vi "App.OpenSequenceSettingsFile.vi"(8 "error in (no error)":errorcluster, 11 "selected path":path) -> (0 "error out":errorcluster, 3 "Settings":T1)   [LabVIEW 2013, in "Simple Sequence Tools - Shared.lvlib"]
uses:
  Simple Sequence Tools - Shared.lvlib
  Types/Saved.Sequence.ctl
  Types/Channel.Properties.ctl
  Main.Constants.vi
  <vilib>/NI/GXML/_subVIs/GXML Quick Parser/Quick Parser.vi
  <vilib>/NI/GXML/GXML.lvlib
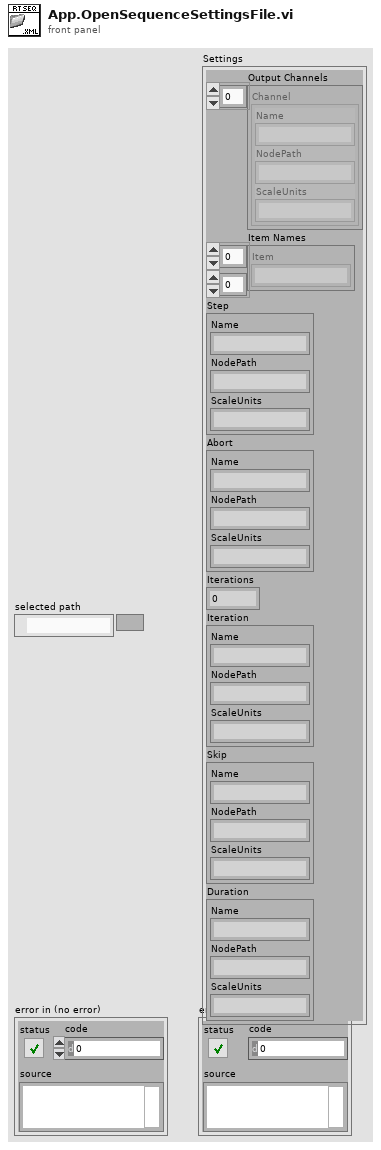
[diagram p1: front panel]
types:
  T1 = typedef "Simple Sequence Tools - Shared.lvlib/Saved.Sequence.ctl" = cluster{"Output Channels":T2[], "Item Names":string[][], "Step":T2, "Abort":T2, "Iterations":u32, "Iteration":T2, "Skip":T2, "Duration":T2}
  T2 = typedef "Simple Sequence Tools - Shared.lvlib/Channel.Properties.ctl" = cluster{"Name":string, "NodePath":string, "ScaleUnits":string}
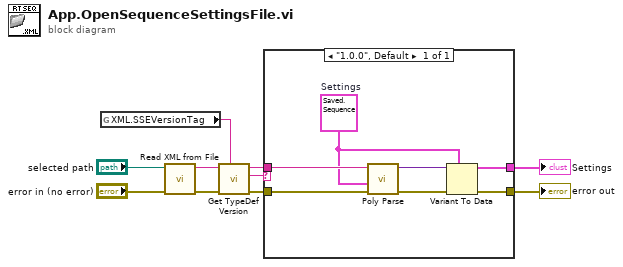
[diagram p0: block diagram]
diagram:
  n1 = global read "Main.Constants.vi" "XML.SSEVersionTag"() -> (w1:string)
  n2 = call <vilib>:"Read XML from File.vi"("error in"="error in (no error)", "XML File Path"="selected path") -> ("error out"=w8:errorcluster, "XML String Out"=w6:string)  [unwired: 8 in]
  n3 = call <vilib>:"Get TypeDef Version.vi"("Version Tag Name"=w1, "error in"=w8, "XML String In"=w6) -> ("error out"=w7:errorcluster, "Version String"=w2:string, "XML String Out"=w5:string)  [unwired: 6 in]
  n4 = case shown="\"1.0.0\", Default" w2 {
    tunnel: w7 -> [w15]
    tunnel: w5 -> [w14]
    tunnel: [w12] -> w4
    tunnel: [w11] -> w3
    frame "1.0.0", Default {
      w13 = T1 {"Output Channels"=[], "Item Names"=[], "Step"={"Name"="", "NodePath"="", "ScaleUnits"=""}, "Abort"={"Name"="", "NodePath"="", "ScaleUnits"=""}, "Iterations"=0, "Iteration"={"Name"="", "NodePath"="", "ScaleUnits"=""}, "Skip"={"Name"="", "NodePath"="", "ScaleUnits"=""}, "Duration"={"Name"="", "NodePath"="", "ScaleUnits"=""}}  # Settings
      n5 = call-poly <vilib>:"Poly Parse.vi"("error in"=w15, "TypeDesc"=w13, "XML File String"=w14) -> ("error out"=w17:errorcluster, "Parsed Data"=w16:variant)  [unwired: 7 in]
      n6 = Variant To Data(error in=w17, type=w13, Variant=w16) -> (data=w12:T1, error out=w11:errorcluster)
    }
  }
  "error out" <- w3
  "Settings" <- w4
